vi "Query Arduino Position.vi"(8 "error in (no error)":errorcluster, 10 "motor (0:n-1)":i32, 11 "VISA resource name":refnum<visa-resource-name>) -> (0 "error out":errorcluster, 1 "pos":i32, 2 "m":i32, 3 "reference out":refnum<visa-resource-name>, 4 "response":string)   [LabVIEW 2024, in "FW Arduino Control.lvclass"]
uses:
  FW Arduino Control.lvclass
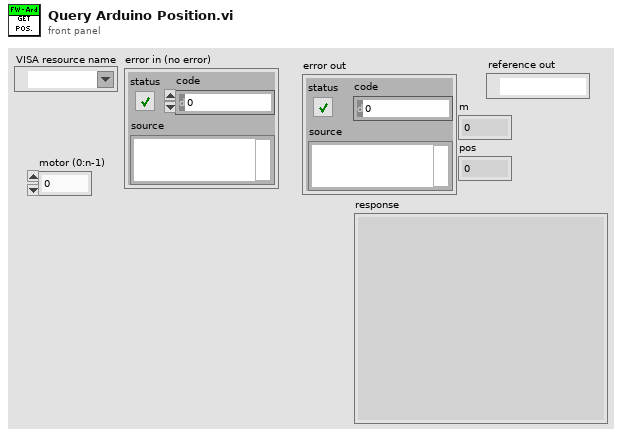
[diagram p1: front panel]
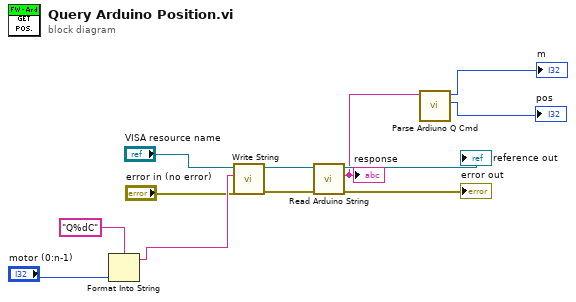
[diagram p0: block diagram]
diagram:
  n1 = Format Into String(format string="Q%dC", "motor (0:n-1)") -> (resulting string=w8:string)  [unwired: 2 in, 1 out]
  n2 = call "Write String.vi"("error in (no error)"="error in (no error)", "String"=w8, "VISA resource name"="VISA resource name") -> ("error out"=w11:errorcluster, "VISA resource name out"=w12:refnum<visa-resource-name>)  [unwired: 7 in]
  n3 = call "Read Arduino String.vi"("error in (no error)"=w11, "reference"=w12) -> ("error out"=→"error out":errorcluster, "response"=w3:string, "reference out"=→"reference out":refnum<visa-resource-name>)  [unwired: 7 in]
  "response" <- w3
  n4 = call "Parse Ardiuno Q Cmd.vi"("Q cmd response"=w3) -> ("pos"=→"pos":i32, "m"=→"m":i32)  [unwired: 8 in, 1 out]
